vi "TCP_receive.vi"(8 "error in (no error)":errorcluster, 10 "queue":refnum<queue>) -> (0 "error out":errorcluster)   [LabVIEW 2013, in "TCP_IP.lvclass"]
uses:
  TCP_IP.lvclass
  Globals.vi
panel:
  out "data out":string
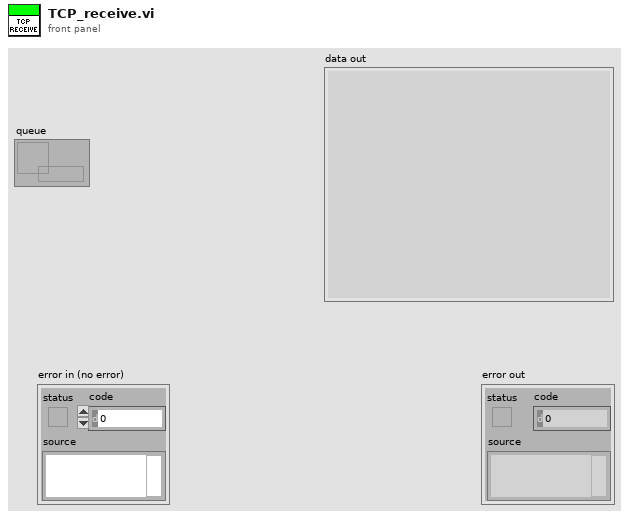
[diagram p1: front panel]
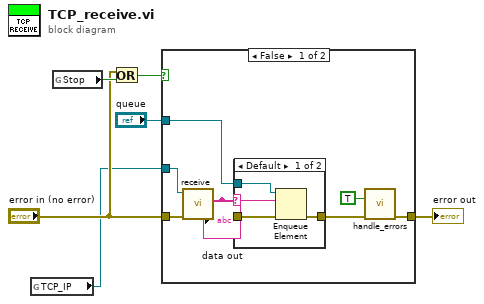
[diagram p0: block diagram]
diagram:
  n1 = global read "Globals.vi" "TCP_IP"() -> (w1:refnum<class "TCP_IP.lvclass">)
  n2 = global read "Globals.vi" "Stop"() -> (w3:bool)
  n3 = Or(x="error in (no error)", y=w3) -> (x .or. y?=w4:bool)
  n4 = case shown="False" w4 {
    tunnel: [w14 w20] -> w6
    tunnel: w1 -> [w8 _]
    tunnel: "queue" -> [w13 _]
    tunnel: "error in (no error)" -> [w9 w20]
    frame False {
      n5 = call "receive.vi"("error in (no error)"=w9, "TCP_IP.lvclass"=w8) -> ("error out"=w11:errorcluster, "data out"=w12:string)  [unwired: 8 in]
      "data out" <- w12
      n6 = case shown="Default" w12 {
        selector: w12 -> [w15 _]
        tunnel: w13 -> [w18 _]
        tunnel: w11 -> [w17 w19]
        tunnel: [w16 w19] -> w10
        frame Default {
          n7 = Enqueue Element(queue=w18, element=w15, error in (no error)=w17) -> (error out=w16:errorcluster)  [unwired: 1 in, 2 out]
        }
        frame "" {
        }
      }
      n8 = call "handle_errors.vi"("Restart Network"=TRUE, "error in (no error)"=w10) -> ("error out"=w14:errorcluster)  [unwired: 13 in]
    }
    frame True {
    }
  }
  "error out" <- w6
